vi "Get Time Since Start.vi"(1 "Start time (s)":dbl format="%.3f", 2 "Accuracy":enum16{"1 ms", "10 ms"}(ring), 3 "Time now (s)":dbl format="%.3f") -> (0 "Difference":dbl format="%.3f")   [LabVIEW 2011]
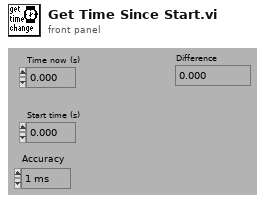
[diagram p1: front panel]
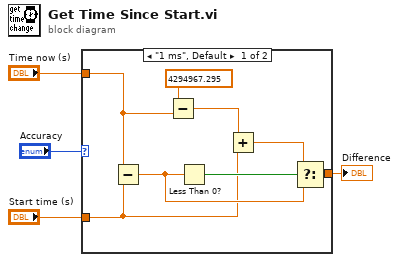
[diagram p0: block diagram]
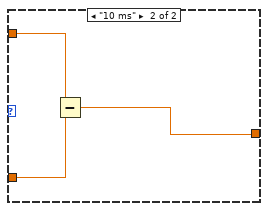
[diagram p2: hidden frame]
diagram:
  n1 = case shown="\"1 ms\", Default" "Accuracy" {
    tunnel: [w12 w13] -> w4
    tunnel: "Time now (s)" -> [w11 w15]
    tunnel: "Start time (s)" -> [w7 w14]
    frame "1 ms", Default {
      n2 = Subtract(x=w11, y=w7) -> (x-y=w10:dbl)
      n3 = Subtract(x=4294967.295, y=w11) -> (x-y=w6:dbl)
      n4 = Less Than 0?(x=w10) -> (x < 0?=w8:bool)
      n5 = Add(x=w6, y=w7) -> (x+y=w9:dbl)
      n6 = Select(t=w9, s=w8, f=w10) -> (s? t:f=w12:dbl)
    }
    frame "10 ms" {
      n7 = Subtract(x=w15, y=w14) -> (x-y=w13:dbl)
    }
  }
  "Difference" <- w4
